vi "Get Cursor Position.vi"(8 "error in (no error)":errorcluster, 10 "Cursor":T1, 11 "PXIe5105 in":refnum<class "PXIe5105.lvclass">) -> (0 "error out":errorcluster, 2 "Position":dbl format="%.9f", 3 "PXIe5105 out":refnum<class "PXIe5105.lvclass">)   [LabVIEW 2018, in "PXIe5105.lvlib" / "PXIe5105.lvclass"]
doc: "This Override method is used to get cursor(s) position from the Oscope instrument. Use 'Cursor' control to select the cursor of interest, and carry out its value to the 'Position' indicator."
uses:
  PXIe5105.lvclass
  PPLs/Oscilloscope/Parent/Oscilloscope.lvlibp/Custom Controls/Select Cursor.ctl
  PPLs/Oscilloscope/Parent/Oscilloscope.lvlibp
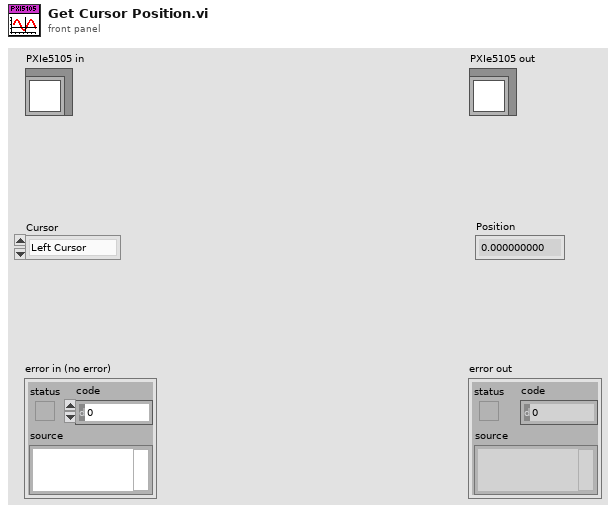
[diagram p1: front panel]
types:
  T1 = typedef "Oscilloscope.lvlibp/Select Cursor.ctl" = enum16{"Left Cursor", "Right Cursor", "Top Cursor", "Bottom Cursor"}
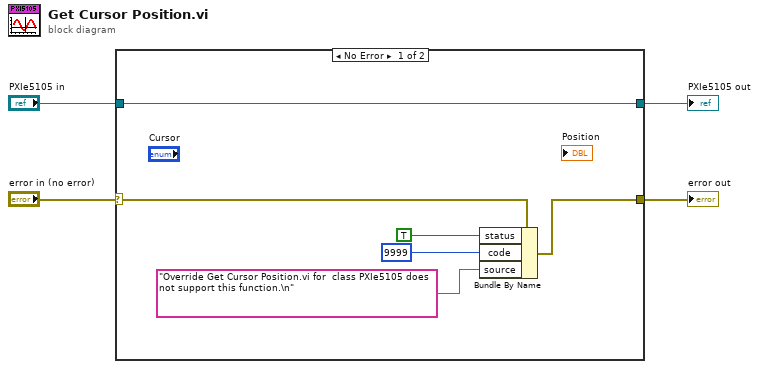
[diagram p0: block diagram]
diagram:
  n1 = case shown="No Error" "error in (no error)" {
    selector: "error in (no error)" -> [w7 w12]
    tunnel: [w6 w12] -> w3
    tunnel: "PXIe5105 in" -> [w5 w11]
    tunnel: [w5 w11] -> w1
    frame No Error {
      n2 = Bundle By Name(cluster=w7, "status"=TRUE, "code"=9999, "source"="Override Get Cursor Position.vi for  class PXIe5105 does not support this function.\n") -> (w6:errorcluster)
    }
    frame Error {
    }
  }
  "error out" <- w3
  "PXIe5105 out" <- w1
